vi "Global.vi"() -> ()   [LabVIEW 2020]
uses:
  controls/Data.ctl
panel:
  out "Act 8":bool
  in  "Ilck 8":bool
  in  "Tr 8":bool
  out "Seq.ui8":T1 caption="UI1"
  out "Act 7":bool
  in  "Ilck 7":bool
  in  "Tr 7":bool
  out "Seq.ui7":T1 caption="UI1"
  out "Act 6":bool
  in  "Ilck 6":bool
  in  "Tr 6":bool
  out "Seq.ui6":T1 caption="UI1"
  out "Act 5":bool
  in  "Ilck 5":bool
  in  "Tr 5":bool
  out "Seq.ui5":T1 caption="UI1"
  out "Act 4":bool
  in  "Ilck 4":bool
  in  "Tr 4":bool
  out "Seq.ui4":T1 caption="UI1"
  out "Act 3":bool
  out "Act 2":bool
  in  "Ilck 3":bool
  in  "Tr 3":bool
  in  "Ilck 2":bool
  in  "Tr 2":bool
  out "Act 1":bool
  in  "Tr 1":bool
  in  "Ilck 1":bool
  out "Seq.ui3":T1 caption="UI1"
  out "Seq.ui2":T1 caption="UI1"
  out "Seq.ui1":T1 caption="UI1"
  out "seq":T3
  # "GENERAL SEQUENCE STRUCTURE"
  # "STEP STRUCTURES (UP TO 8 STEP, BUT COULD BE ADDED MORE)"
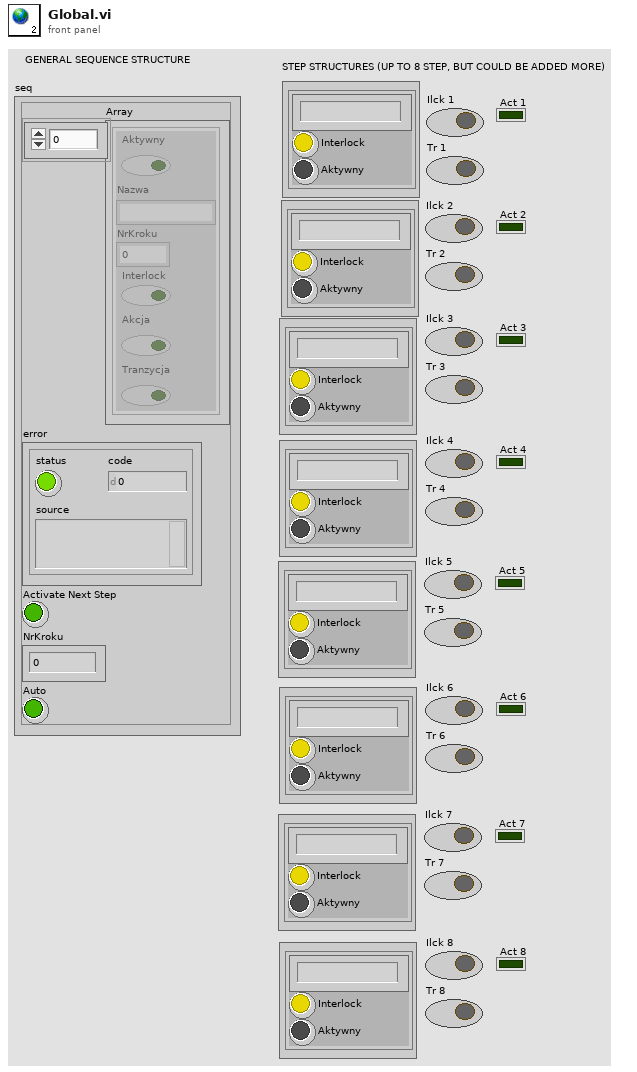
[diagram p1: front panel]
types:
  T1 = cluster{string, "Interlock":bool, "Aktywny":bool}
  T2 = typedef "Data.ctl" = cluster{"Aktywny":bool, "Nazwa":string, "NrKroku":dbl, "Interlock":bool, "Akcja":bool, "Tranzycja":bool}
  T3 = cluster{"Array":T2[], "error":errorcluster, "Activate Next Step":bool, "NrKroku":dbl, "Auto":bool}
diagram:
